vi "Serialize.vi"(8 "error in (no error)":errorcluster, 10 "Element in":refnum<k20>, 11 "Test Case in":refnum<class "Test Case.lvclass">) -> (0 "error out":errorcluster, 2 "Element out":refnum<k20>)   [LabVIEW 2013, in "JUnit XML.lvlib" / "Test Case.lvclass"]
doc: "Serializes a Test Case using NI XML Parser."
uses:
  Test Case.lvclass
  Test Case.lvclass/Test Case.ctl
  <vilib>/xml/Close Reference(Node).vi
  <vilib>/xml/NI_XML.lvlib
  JUnit XML.lvlib
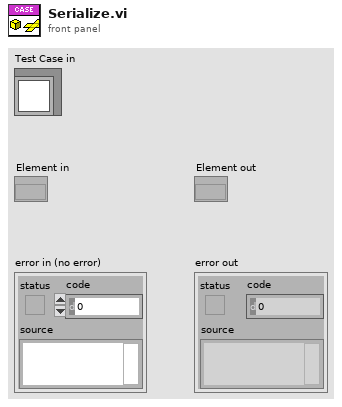
[diagram p1: front panel]
types:
  T1 = typedef "JUnit XML.lvlib/Test Case.lvclass/Test Result.ctl" = enum16{"Success", "Failure", "Error", "Skipped"}
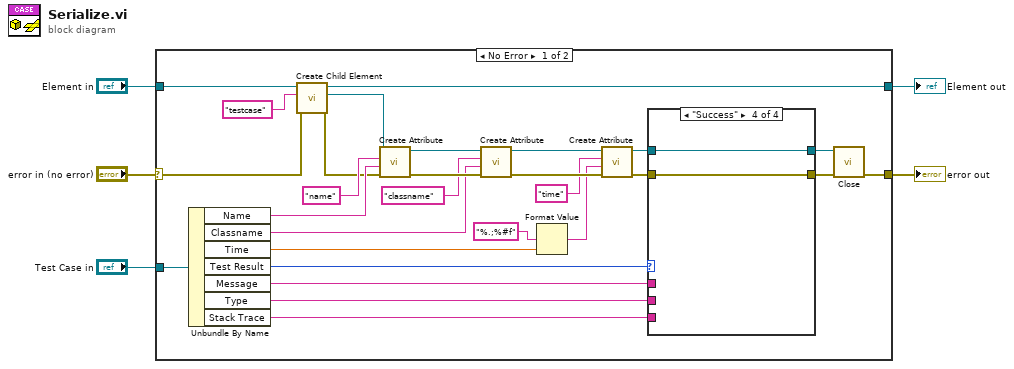
[diagram p0: block diagram]
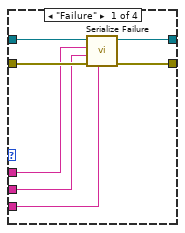
[diagram p2: hidden frame]
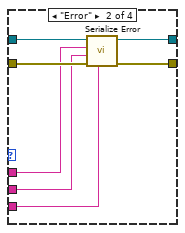
[diagram p3: hidden frame]
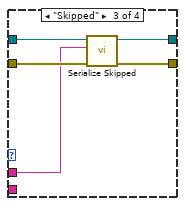
[diagram p4: hidden frame]
diagram:
  n1 = case shown="No Error" "error in (no error)" {
    selector: "error in (no error)" -> [w10 w56]
    tunnel: [w9 w56] -> w4
    tunnel: "Test Case in" -> [w8 _]
    tunnel: "Element in" -> [w7 w55]
    tunnel: [w6 w55] -> w1
    frame No Error {
      n2 = Unbundle By Name(w8) -> ("Name"=w31:string, "Classname"=w21:string, "Time"=w20:dbl, "Test Result"=w18:T1, "Message"=w15:string, "Type"=w14:string, "Stack Trace"=w11:string)
      n3 = call "Create Child Element.vi"("error in (no error)"=w10, "Name"="testcase" ("Tag Name"), "Element in"=w7) -> ("error out"=w22:errorcluster, "Child Element"=w23:refnum<k20>, "Element out"=w6:refnum<k20>)  [unwired: 6 in]
      n4 = call "Create Attribute.vi"("error in (no error)"=w22, "Value"=w31, "Name"="name" ("Attribute Name"), "Element in"=w23) -> ("error out"=w29:errorcluster, "Element out"=w30:refnum<k20>)  [unwired: 6 in]
      n5 = call "Create Attribute.vi"("error in (no error)"=w29, "Value"=w21, "Name"="classname" ("Attribute Name"), "Element in"=w30) -> ("error out"=w26:errorcluster, "Element out"=w27:refnum<k20>)  [unwired: 6 in]
      n6 = Format Value(format string="%.;%#f", value (0)=w20) -> (output string=w19:string)  [unwired: 1 in]
      n7 = call "Create Attribute.vi"("error in (no error)"=w26, "Value"=w19, "Name"="time" ("Attribute Name"), "Element in"=w27) -> ("error out"=w12:errorcluster, "Element out"=w13:refnum<k20>)  [unwired: 6 in]
      n8 = case shown="\"Success\"" w18 {
        tunnel: w13 -> [w40 w47 w52 w54]
        tunnel: [w39 w46 w51 w54] -> w17
        tunnel: [w38 w45 w50 w53] -> w16
        tunnel: w12 -> [w37 w44 w49 w53]
        tunnel: w15 -> [w36 w43 w48 _]
        tunnel: w14 -> [w35 w42 _ _]
        tunnel: w11 -> [w34 w41 _ _]
        frame "Failure" {
          n9 = call "Serialize Failure.vi"("Stack Trace"=w34, "error in (no error)"=w37, "Type"=w35, "Message"=w36, "Node in"=w40) -> ("error out"=w38:errorcluster, "Node out"=w39:refnum<k20>)  [unwired: 5 in]
        }
        frame "Error" {
          n10 = call "Serialize Error.vi"("Stack Trace"=w41, "error in (no error)"=w44, "Type"=w42, "Message"=w43, "Node in"=w47) -> ("error out"=w45:errorcluster, "Node out"=w46:refnum<k20>)  [unwired: 5 in]
        }
        frame "Skipped" {
          n11 = call "Serialize Skipped.vi"("error in (no error)"=w49, "Message"=w48, "Node in"=w52) -> ("error out"=w50:errorcluster, "Node out"=w51:refnum<k20>)  [unwired: 7 in]
        }
        frame "Success" {
        }
      }
      n12 = call-poly <vilib>:"Close.vi"("error in (no error)"=w16, "node"=w17) -> ("error out"=w9:errorcluster)  [unwired: 7 in]
    }
    frame Error {
    }
  }
  "error out" <- w4
  "Element out" <- w1
